vi "NearWaypointTest.vi"(8 "Yrobot":dbl, 9 "Xrobot":dbl, 10 "Ywaypoint":dbl, 11 "Xwaypoiny":dbl) -> (2 "AtWaypoint":bool)   [LabVIEW 2012]
doc: "This VI checks to see if the robots curretn position is close to the next waypoint. If it is, it sets a boolean flag to allow a case statement to update the MDF"
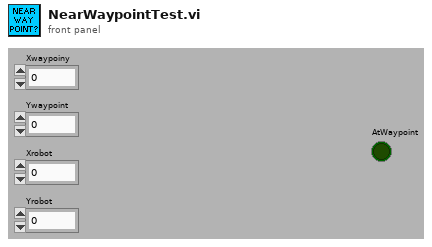
[diagram p1: front panel]
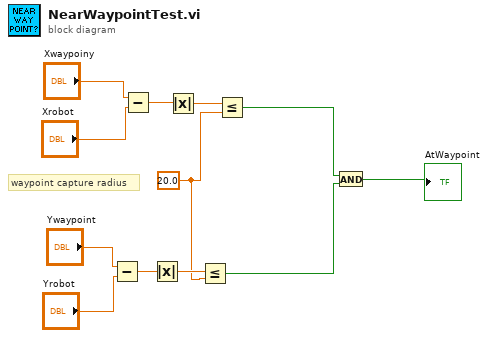
[diagram p0: block diagram]
diagram:
  w4 = 20.0 ("y")
  # "waypoint capture radius"
  n1 = Subtract(x="Ywaypoint", y="Yrobot") -> (x-y=w7:dbl)
  n2 = Subtract(x="Xwaypoiny", y="Xrobot") -> (x-y=w8:dbl)
  n3 = Absolute Value(x=w7) -> (abs(x)=w6:dbl)
  n4 = Absolute Value(x=w8) -> (abs(x)=w5:dbl)
  n5 = Less Or Equal?(x=w6, y=w4) -> (x <= y?=w2:bool)
  n6 = Less Or Equal?(x=w5, y=w4) -> (x <= y?=w3:bool)
  n7 = And(x=w3, y=w2) -> (x .and. y?=→"AtWaypoint":bool)
